vi "Test DRAM Throughput_pipelined.vi"(7 "fifo depth":u8(ring)=16 items=["4"=2, "8"=3, "16"=4, "32"=5, "64"=6, "128"=7, "256"=8, "512"=9, "1024"=10, "2048"=11, "4096"=12, "8192"=13, "16384"=14, "32768"=15, "65536"=16, "131072"=17, "262144"=18, "524288"=19, "1048576"=20, "2097152"=21, "4194304"=22, "8388608"=23, "16777216"=24, "33554432"=25, "67108864"=26, "134217728"=27, "268435456"=28, "536870912"=29, "1073741824"=30, "2147483648"=31, "4294967296"=32], 10 "arbiter configuration":T3={"write grant time (clocks)"=100, "read grant time (clocks)"=100}, 11 "Points to Generate":u32=100 format="%.0p") -> (2 "Pass?":bool, 3 "Write Throughput (Bytes/sec)":u32 format="%.2p")   [LabVIEW 2011]
uses:
  <instrlib>/FlexRIO/Libraries/Memory/FPGA/Interface/Timeslot Arbiter Configuration.ctl
  <instrlib>/RF-RIO/FIFO/FIFO/FPGA/Public/FIFO State.ctl
  <vilib>/Platform/TimedLoop/XDataNode/timing_clust.ctl
  <vilib>/Platform/TimedLoop/XDataNode/nitl_modes.ctl
  <vilib>/Platform/TimedLoop/XDataNode/wakeup.ctl
  <vilib>/Platform/TimedLoop/XDataNode/XDataNode.xnode
  <vilib>/rvi/FXPMathLib/basic elements/FxpDiscreteDelay/XNode/nifxpmath_DiscreteDelay.xnode
  <instrlib>/RF-RIO/FIFO/FIFO/FPGA/FIFO.lvlib
  <vilib>/Platform/TimedLoop/XDataNode/XDNodeRunTimeDep.lvlib
  <instrlib>/FlexRIO/Libraries/Memory/FPGA/Memory.lvlib
panel:
  out "Generation Done Ticks":i32
  out "DRAM Retrieval in Ticks":u32
  out "count 2":u32
  out "state":T1
  out "count":u32
  out "bank1.data":T2
  out "bank0.data":T2
  out "Last Address Failed":u32
  out "Points Read from FIFO":u32
  out "Read Throughput (Bytes/sec)":u32 format="%.2p"
  out "Gen. Points Done":u32 format="%.0p"
  out "Generation Done?":bool
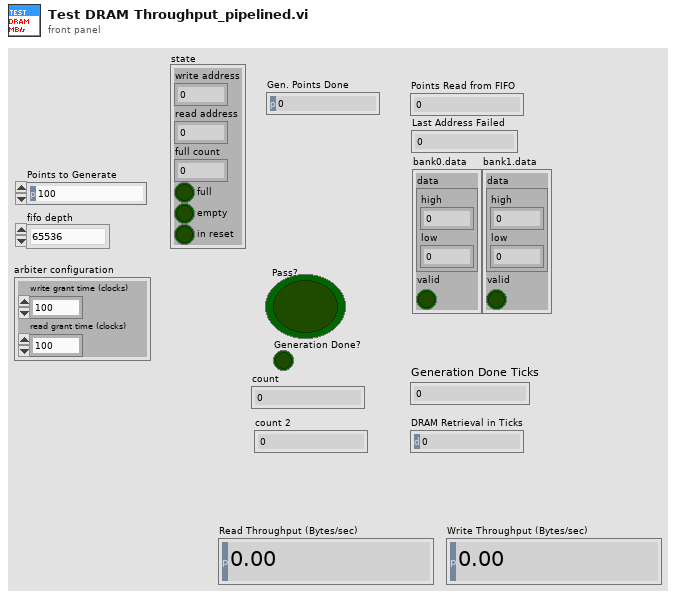
[diagram p1: front panel]
types:
  T1 = typedef "FIFO.lvlib/FIFO State.ctl" = cluster{"write address":u32, "read address":u32, "full count":u32, "full":bool, "empty":bool, "in reset":bool}
  T2 = cluster{"data":cluster{"high":u64, "low":u64}, "valid":bool}
  T3 = typedef "Memory.lvlib/Timeslot Arbiter Configuration.ctl" = cluster{"write grant time (clocks)":u16, "read grant time (clocks)":u16}
  T4 = typedef "XDNodeRunTimeDep.lvlib/timing_clust.ctl" = cluster{"Expected End [f-1]":u64, "Actual End [f-1]":u64, "Finished Late? [f-1]":bool, "Expected End [i-1]":u64, "Actual End [i-1]":u64, "Finished Late? [i-1]":bool, "Expected Start [i]":u64, "Actual Start [i]":u64, "Expected Start [f]":u64, "Actual Start [f]":u64, "Source Name":string, "Structure Name":string, "Period":i64, "Deadline":i64, "Offset":i64, "Start":i64, "Priority":i32, "Timeout":i32, "Mode":T5, "Wakeup Reason":T6, "Error":errorcluster, "Source Type":string, "Secondary Source Type":string, "Global End Time":u64, "Global Start Time":u64, "Frame Duration":u64, "Iteration Duration":u64, "Assigned CPU":i32, "I/O Scan Engine Mode":u32}
  T5 = typedef "XDNodeRunTimeDep.lvlib/nitl_modes.ctl" = enum32{"No Change", "Process missed periods, maintain original phase", "Discard missed periods, maintain original phase", "Process missed periods, ignore original phase", "Discard missed periods, ignore original phase"}
  T6 = typedef "XDNodeRunTimeDep.lvlib/wakeup.ctl" = enum32{"Normal", "Aborted", "Asynchronous wakeup", "Timing source error", "Timed loop error", "Timeout"}
  T7 = cluster{"fifo1 memory":refnum<k21>, "fifo2 memory":refnum<k21>}
  T8 = typedef "Data Type (256).ctl" = cluster{"Bank0. High":u64, "Bank0. Low":u64, "Bank1. High":u64, "Bank1. Low":u64}
  T9 = cluster{"Bank0. High":u64, "Bank0. Low":u64, "Bank1. High":u64, "Bank1. Low":u64}
  T10 = typedef "FIFO.lvlib/niRFRIO Memory 1.0.0 FPGA.lvlib/Retrieve Data (128-Bit).ctl" = cluster{"data":T11, "valid":bool}
  T11 = typedef "FIFO.lvlib/niRFRIO Memory 1.0.0 FPGA.lvlib/U128.ctl" = cluster{"high":u64, "low":u64}
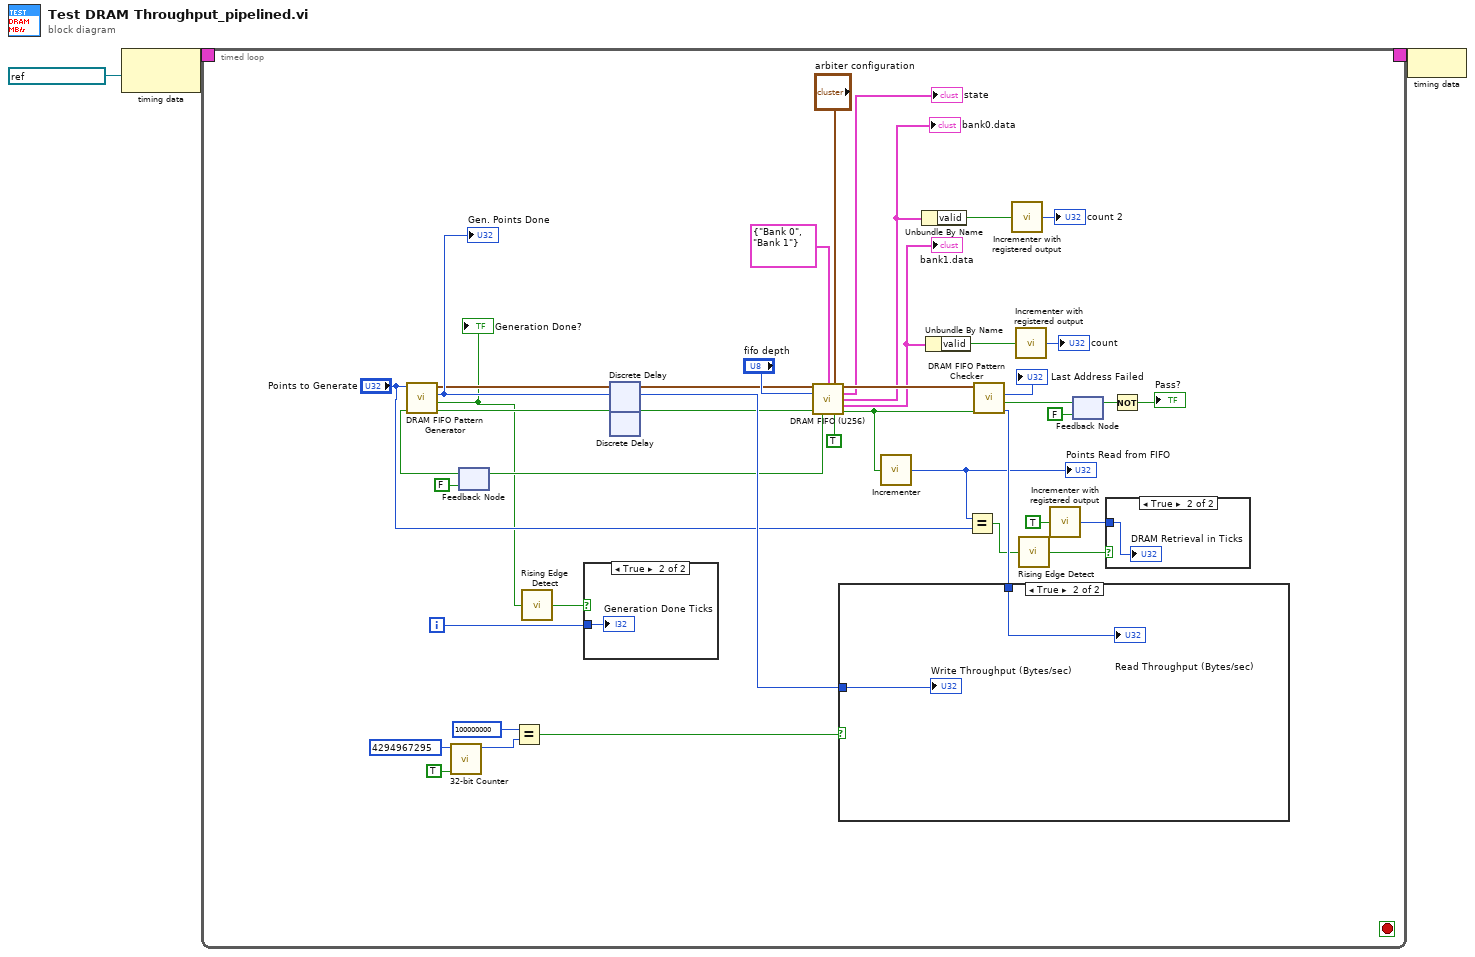
[diagram p0: block diagram]
diagram:
  n1 = node-c288(refnum<k21> "100 MHz Clock" ("Source Name")) -> (w3:T4)
  n2 = timed-loop {
    timing: w3 -> [_]
    timing-out: [_] -> w2
    i -> [w8]
    stop <- _ stop-if-true
    n3 = call <userlib>:"32-bit Counter.vi"("INC?"=TRUE, "rollover"=u32 4294967295) -> ("count"=w33:u32)  [unwired: 9 in]
    n4 = feedback #1(FALSE ("Ready for Input")) -> (w43:bool)
    n5 = call <userlib>:"DRAM FIFO Pattern Generator.vi"("Generate Point"=w43, "Points to Generate"="Points to Generate") -> ("Output Valid"=w9:bool, "Generation Done?"=w7:bool, "Points Done"=w29:u32, "Output Data"=w20:T8)  [unwired: 6 in]
    "Generation Done?" <- w7
    "Gen. Points Done" <- w29
    n6 = Equal?(x=u32 100000000, y=w33) -> (x = y?=w34:bool)
    n7 = call <userlib>:"Rising Edge Detect.vi"("signal"=w7) -> ("edge detected"=w6:bool)  [unwired: 14 in]
    n8 = case shown="True" w6 {
      tunnel: w8 -> [_ w45]
      frame False {
      }
      frame True {
        "Generation Done Ticks" <- w45
      }
    }
    n9 = xnode "Discrete Delay"("D"=w20) -> ("Q"=w5:T9)
    n10 = xnode "Discrete Delay"("D"=w9) -> ("Q"=w4:bool)
    n11 = call <userlib>:"DRAM FIFO (U256).vi"("Input Data"=w5, "Memory"=T7 {"fifo1 memory"="Bank 0", "fifo2 memory"="Bank 1"}, "arbiter configuration"="arbiter configuration", "fifo depth"="fifo depth", "input valid"=w4, "ready for output"=TRUE) -> ("Output Data"=w37:T8, "state"=→"state":T1, "bank0.data"=w18:T10, "Bank1.data"=w16:T10, "Ready for Input"=w27:bool, "Output Valid"=w25:bool)  [unwired: 4 in]
    "bank0.data" <- w18
    "bank1.data" <- w16
    n12 = feedback-in #1(w27) -> ()
    n13 = call <userlib>:"Incrementer.vi"("INC?"=w25) -> ("count"=w15:u32)  [unwired: 4 in]
    "Points Read from FIFO" <- w15
    n14 = Unbundle By Name(w18) -> ("valid"=w19:bool)
    n15 = Unbundle By Name(w16) -> ("valid"=w17:bool)
    n16 = Equal?(x=w15, y="Points to Generate") -> (x = y?=w11:bool)
    n17 = call <userlib>:"DRAM FIFO Pattern Checker.vi"("Input Valid"=w25, "Input Data"=w37) -> ("Points Done"=w28:u32, "Pattern Match Ever Fail?"=w42:bool, "Last Address Failed"=→"Last Address Failed":u32)  [unwired: 3 in, 4 out]
    n18 = case shown="True" w34 {
      tunnel: w29 -> [_ w48]
      tunnel: w28 -> [_ w47]
      frame False {
      }
      frame True {
        "Write Throughput (Bytes/sec)" <- w48
        "Read Throughput (Bytes/sec)" <- w47
      }
    }
    n19 = call <userlib>:"Incrementer with registered output.vi"("INC?"=w19) -> ("count"=→"count 2":u32)  [unwired: 4 in]
    n20 = call <userlib>:"Incrementer with registered output.vi"("INC?"=w17) -> ("count"=→"count":u32)  [unwired: 4 in]
    n21 = call <userlib>:"Rising Edge Detect.vi"("signal"=w11) -> ("edge detected"=w10:bool)  [unwired: 14 in]
    n22 = call <userlib>:"Incrementer with registered output.vi"("INC?"=TRUE) -> ("count"=w13:u32)  [unwired: 4 in]
    n23 = feedback #2(FALSE ("Pattern Match Ever Fail?")) -> (w36:bool)
    n24 = feedback-in #2(w42) -> ()
    n25 = case shown="True" w10 {
      tunnel: w13 -> [_ w46]
      frame False {
      }
      frame True {
        "DRAM Retrieval in Ticks" <- w46
      }
    }
    n26 = Not(x=w36) -> (.not. x?=→"Pass?":bool)
  }
  n27 = node-c288(w2) -> ()
